vi "armctrl-arm-system-simulation-init.vi"() -> (1 "SingleJointArmSim":T3 {"GearBox"."Jr_KgM2" format="%13.5p"; "GearBox"."L_H" format="%13.5p"; "GearBox"."Kt_NMPerAmp" format="%13.5p"; "GearBox"."KvINV_RadPerSecPerVolt" format="%13.5p"; "GearBox"."R_Ohms" format="%13.5p"; "GearBox"."FreeSpeed_RadPerSec" format="%13.5p"; "GearBox"."FreeCurrent_Amps" format="%13.5p"; "GearBox"."StallCurrent_Amps" format="%13.5p"; "GearBox"."StallTorque_NM" format="%13.5p"; "GearBox"."nominalVoltage_Volts" format="%13.5p"}, 2 "Linearsystem":T1, 3 "DCMOTOR":T5 {"Jr_KgM2" format="%13.5p"; "L_H" format="%13.5p"; "Kt_NMPerAmp" format="%13.5p"; "KvINV_RadPerSecPerVolt" format="%13.5p"; "R_Ohms" format="%13.5p"; "FreeSpeed_RadPerSec" format="%13.5p"; "FreeCurrent_Amps" format="%13.5p"; "StallCurrent_Amps" format="%13.5p"; "StallTorque_NM" format="%13.5p"; "nominalVoltage_Volts" format="%13.5p"})   [LabVIEW 2019]
uses:
  <vilib>/Rock Robotics/WPI/ThirdParty/JAS_Junk/TrajLib/Trajectory_Library.lvlib
  <vilib>/Rock Robotics/WPI/ThirdParty/JAS_Junk/TrajLib/DCMotor_GetNEO.vi
  <vilib>/Rock Robotics/WPI/ThirdParty/JAS_Junk/TrajLib/TypeDef/DCMOTOR.CTL
  <vilib>/Analysis/Matrix/Datatypes/RealMatrix.ctl
  <vilib>/Analysis/Matrix/NI_Matrix.lvlib
  <vilib>/Rock Robotics/WPI/ThirdParty/JAS_Junk/TrajLib/TypeDef/LINEAR_SYSTEM.ctl
  <vilib>/Rock Robotics/WPI/ThirdParty/JAS_Junk/TrajLib/TypeDef/LINEAR_SYSTEM_SIM.ctl
  <vilib>/Rock Robotics/WPI/ThirdParty/JAS_Junk/TrajLib/TypeDef/SINGLE_JOINT_ARM_SIM.ctl
panel:
  # "<States,States>"
  # "<States,Inputs>"
  # "<Outputs,States>"
  # "<Outputs,Inputs>"
  # "<States, 1>"
  # "<Outputs, 1>"
  # "<Inputs, 1>"
  # "<Outputs, 1>"
  # "<States,States>"
  # "<States,Inputs>"
  # "<Outputs,States>"
  # "<Outputs,Inputs>"
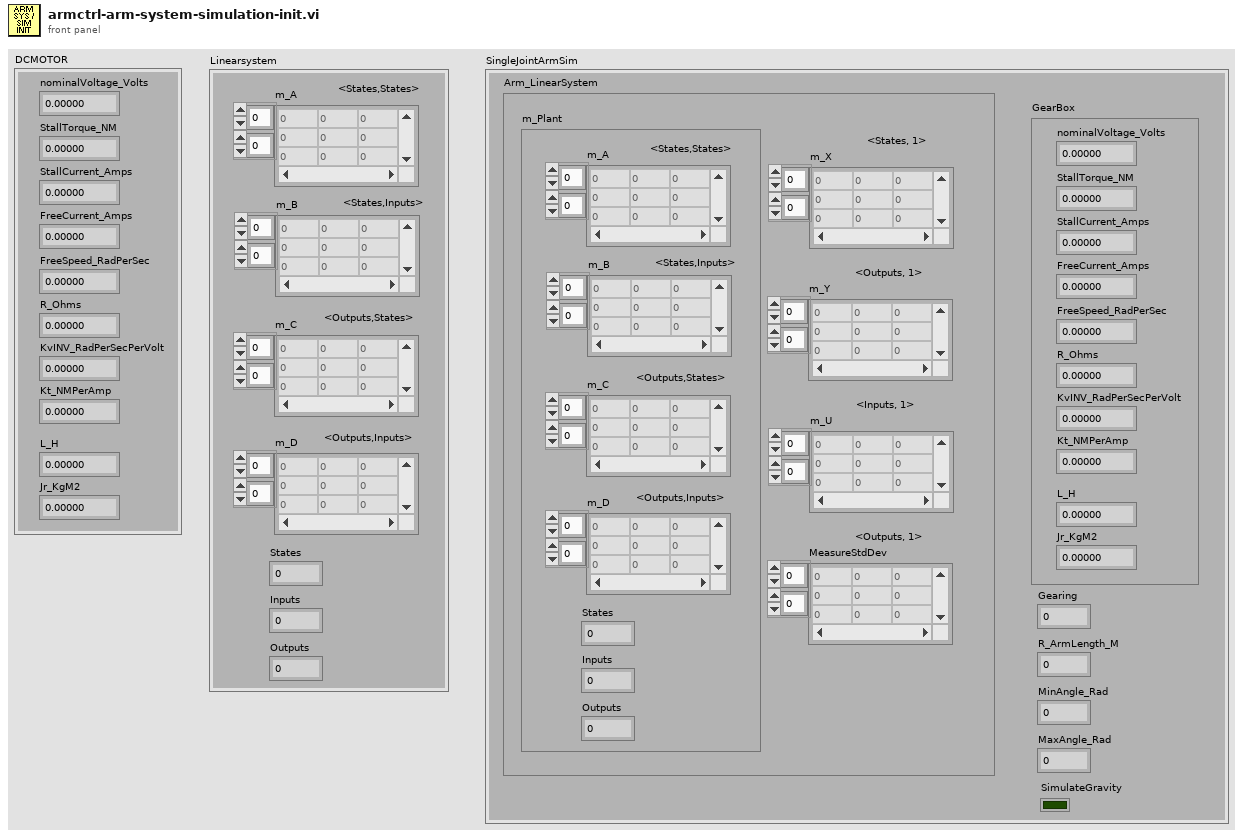
[diagram p1: front panel]
types:
  T1 = typedef "Trajectory_Library.lvlib/LINEAR_SYSTEM.ctl" = cluster{"m_A":T2, "m_B":T2, "m_C":T2, "m_D":T2, "States":i32, "Inputs":i32, "Outputs":i32}
  T2 = typedef "NI_Matrix.lvlib/RealMatrix.ctl" = dbl[][]
  T3 = typedef "Trajectory_Library.lvlib/SINGLE_JOINT_ARM_SIM.ctl" = cluster{"Arm_LinearSystem":T4, "GearBox":T5, "Gearing":dbl, "R_ArmLength_M":dbl, "MinAngle_Rad":dbl, "MaxAngle_Rad":dbl, "SimulateGravity":bool}
  T4 = typedef "Trajectory_Library.lvlib/LINEAR_SYSTEM_SIM.ctl" = cluster{"m_Plant":T1, "m_X":T2, "m_Y":T2, "m_U":T2, "MeasureStdDev":T2}
  T5 = typedef "Trajectory_Library.lvlib/DCMOTOR.CTL" = cluster{"nominalVoltage_Volts":dbl, "StallTorque_NM":dbl, "StallCurrent_Amps":dbl, "FreeCurrent_Amps":dbl, "FreeSpeed_RadPerSec":dbl, "R_Ohms":dbl, "KvINV_RadPerSecPerVolt":dbl, "Kt_NMPerAmp":dbl, "L_H":dbl, "Jr_KgM2":dbl}
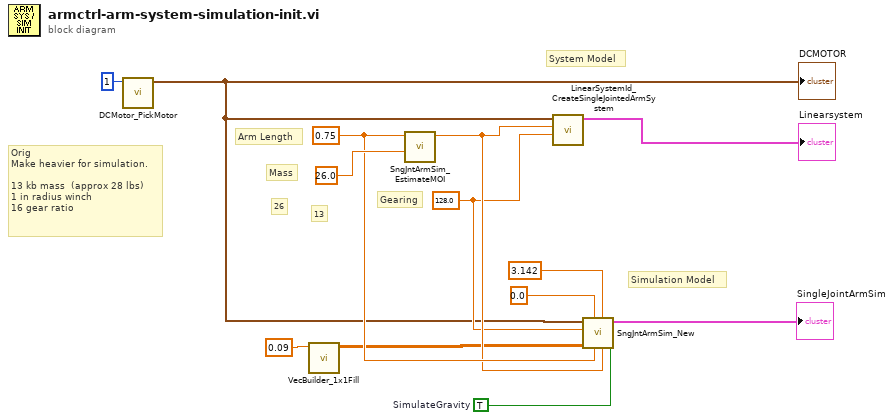
[diagram p0: block diagram]
diagram:
  w13 = TRUE  # SimulateGravity
  w11 = 0.75 ("ArmLength_M")
  w8 = 128.0 ("G")
  # "26"
  # "13"
  # "Simulation Model"
  # "System Model"
  # "Arm Length"
  # "Mass"
  # "Orig\nMake heavier for simulation.\n\n13 kb mass  (approx 28 lbs)\n1 in radius winch\n16 gear ratio"
  # "Gearing"
  n1 = call-poly <vilib>:"DCMotor_PickMotor.vi"("Num Motors"=1) -> ("DCMOTOR"=w5:T5)  [unwired: 10 in]
  "DCMOTOR" <- w5
  n2 = call <vilib>:"VecBuilder_1x1Fill.vi"("R0_C0"=0.09) -> ("output matrix"=w9:T2)  [unwired: 10 in]
  n3 = call <vilib>:"SngJntArmSim_EstimateMOI.vi"("ArmMass_Kg"=26.0 ("massKg"), "ArmLength_M"=w11) -> ("MOI"=w10:dbl)  [unwired: 9 in]
  n4 = call <vilib>:"LinearSystemId_CreateSingleJointedArmSystem.vi"("G"=w8, "jKgSquaredMeters"=w10, "DCMOTOR"=w5) -> ("Linearsystem"=→"Linearsystem":T1)  [unwired: 7 in, 1 out]
  n5 = call <vilib>:"SngJntArmSim_New.vi"("SimulateGravity"=w13, "jKgMetersSquared"=w10, "MaxAngle_Rad"=3.142 ("MaxHeight_Meters"), "ArmLength_Meters"=w11, "MinAngle_Rad"=0.0 ("MinHeight_Meters"), "MeasurementStdDev"=w9, "Gearing"=w8, "GearBox"=w5) -> ("SingleJointArmSim"=→"SingleJointArmSim":T3)  [unwired: 2 in, 1 out]
